vi "matched_filtering.vi"(8 "error in (no error)":errorcluster, 10 "input complex waveform":cluster{"t0":dbl, "dt":dbl, "Y":cdb[]}, 11 "Modulation Parameters In":T1={"RX Parameters"={"RX Oversample Factor"=4, "RX Sample Rate"=4000000.0, "Synchronization Options"={"Synchronization Method"=enum."Fixed Offset", "Symbol Timing Recovery Method "=enum."MT Allign To Ideal Symbols", "Fixed Offset"=0.0, "Frame Detection Method"=enum."", "Correct Frequency Offset"=FALSE}, "Channel Estimation/Equalization Parameters"={"Equalization Method"=enum."", "Channel Estimate Length"=0.0, "Equalizer Length"=0.0, "Equalizer Delay"=0.0}}, "TX/RX Shared Parameters"={"Modulation Type"=enum."OOK", "Packet Length"=128, "# of Iterations"=0.0, "Pulse Shaping Parameters"={"Pulse Shaping Filter"=enum."none", "Filter Length (symbols)"=32, "Filter Parameter"=0.8, "modulation type"=enum."FSK"}, "Header/Tail Control Information"={"Training Sequence Type"=enum."", "Zero Pad Length"=0.0}}}) -> (0 "error out":errorcluster, 2 "output complex waveform":cluster{"t0":dbl, "dt":dbl, "Y":cdb[]}, 3 "Modulation Parameters Out":T1={"RX Parameters"={"RX Oversample Factor"=4, "RX Sample Rate"=4000000.0, "Synchronization Options"={"Synchronization Method"=enum."Fixed Offset", "Symbol Timing Recovery Method "=enum."MT Allign To Ideal Symbols", "Fixed Offset"=0.0, "Frame Detection Method"=enum."", "Correct Frequency Offset"=FALSE}, "Channel Estimation/Equalization Parameters"={"Equalization Method"=enum."", "Channel Estimate Length"=0.0, "Equalizer Length"=0.0, "Equalizer Delay"=0.0}}, "TX/RX Shared Parameters"={"Modulation Type"=enum."OOK", "Packet Length"=128, "# of Iterations"=0.0, "Pulse Shaping Parameters"={"Pulse Shaping Filter"=enum."none", "Filter Length (symbols)"=32, "Filter Parameter"=0.8, "modulation type"=enum."FSK"}, "Header/Tail Control Information"={"Training Sequence Type"=enum."", "Zero Pad Length"=0.0}}})   [LabVIEW 2012]
uses:
  <vilib>/Analysis/2dsp.llb/1D Convolution (CDB).vi
  <vilib>/addons/Modulation/niDMT.lvlib
  <vilib>/Analysis/NI_AALPro.lvlib
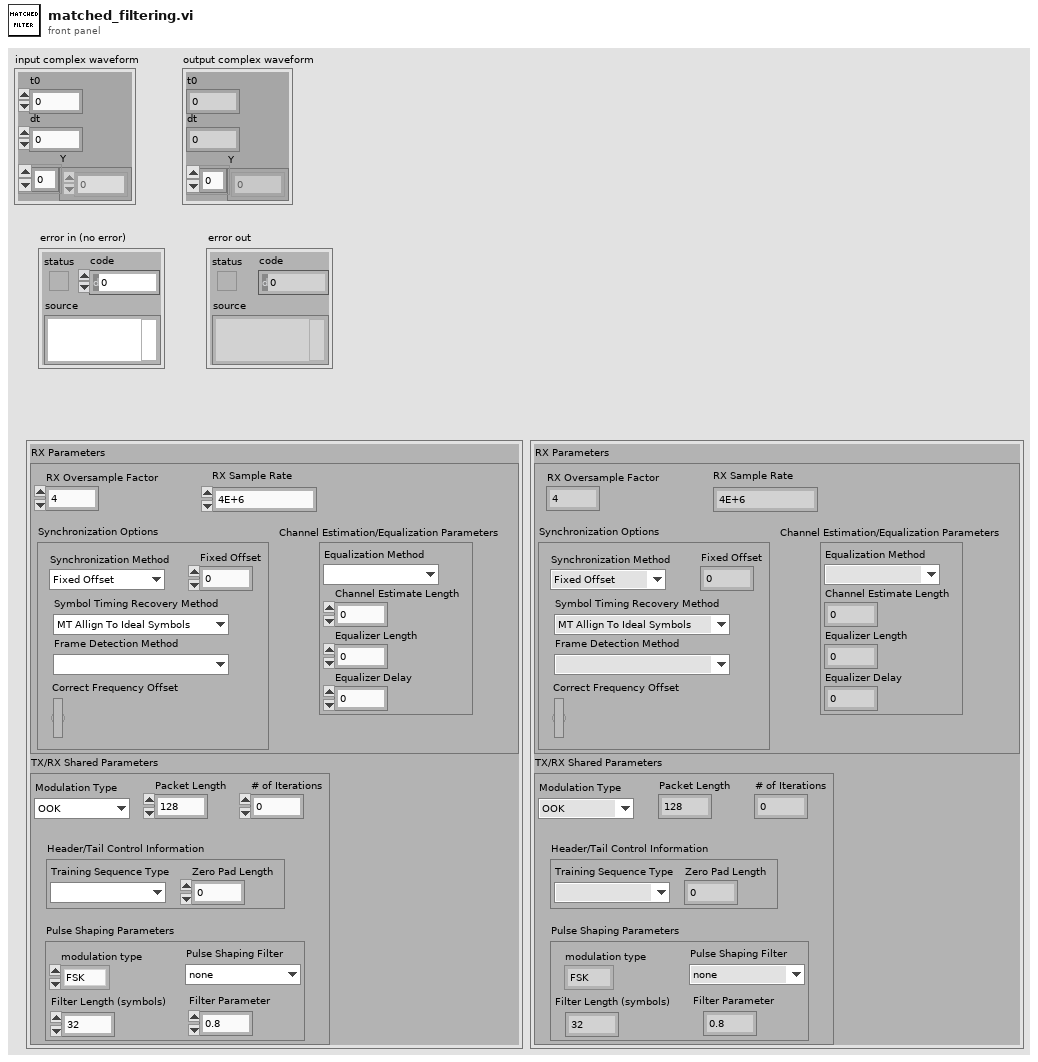
[diagram p1: front panel]
types:
  T1 = cluster{"RX Parameters":cluster{"RX Oversample Factor":i32, "RX Sample Rate":dbl, "Synchronization Options":cluster{"Synchronization Method":enum16{"Fixed Offset", "Timing Estimation", "Joint Timing and Channel Estimation"}, "Symbol Timing Recovery Method ":enum16{"MT Allign To Ideal Symbols", "Maximum Energy", "Early-Late Gate", "Gardner", "Fixed Offset"}, "Fixed Offset":dbl, "Frame Detection Method":enum16{""}, "Correct Frequency Offset":bool}, "Channel Estimation/Equalization Parameters":cluster{"Equalization Method":enum16{""}, "Channel Estimate Length":dbl, "Equalizer Length":dbl, "Equalizer Delay":dbl}}, "TX/RX Shared Parameters":cluster{"Modulation Type":enum16{"OOK", "FSK"}, "Packet Length":i32, "# of Iterations":dbl, "Pulse Shaping Parameters":cluster{"Pulse Shaping Filter":enum16{"none", "Raised Cosine", "Root Raised Cos", "Gaussian"}, "Filter Length (symbols)":i32, "Filter Parameter":dbl, "modulation type":enum16{"FSK", "PSK", "QAM", "MSK", "PAM", "ASK", "CPM"}}, "Header/Tail Control Information":cluster{"Training Sequence Type":enum16{""}, "Zero Pad Length":dbl}}}
  T2 = cluster{"Pulse Shaping Filter":enum16{"none", "Raised Cosine", "Root Raised Cos", "Gaussian"}, "Filter Length (symbols)":i32, "Filter Parameter":dbl, "modulation type":enum16{"FSK", "PSK", "QAM", "MSK", "PAM", "ASK", "CPM"}}
  T3 = enum16{"FSK", "PSK", "QAM", "MSK", "PAM", "ASK", "CPM"}
  T4 = enum16{"none", "Raised Cosine", "Root Raised Cos", "Gaussian"}
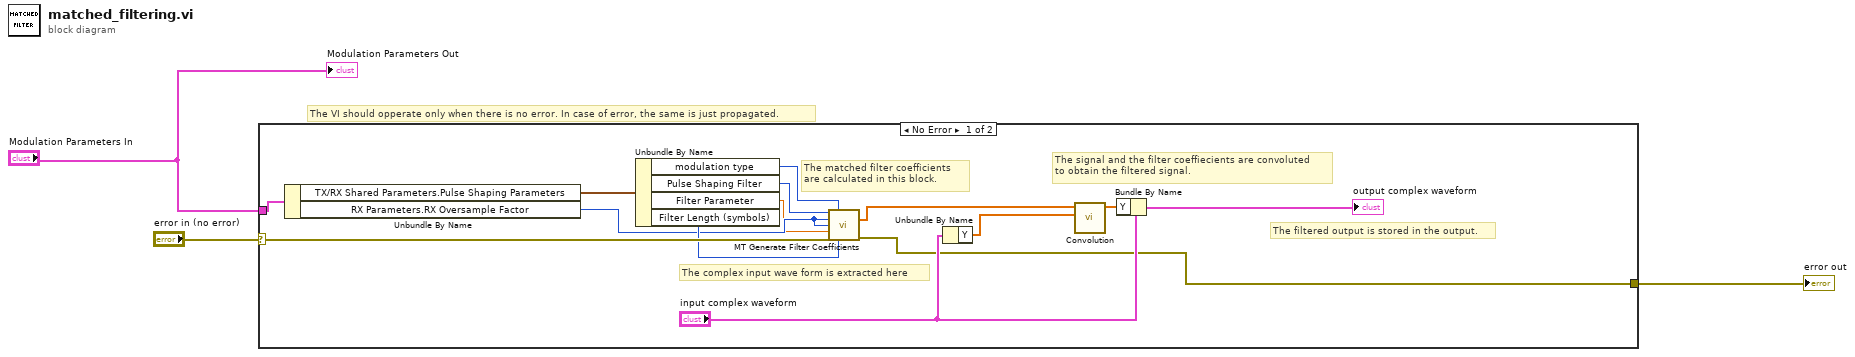
[diagram p0: block diagram]
diagram:
  # "The VI should opperate only when there is no error. In case of error, the same is just propagated."
  n1 = case shown="No Error" "error in (no error)" {
    selector: "error in (no error)" -> [w15 w18]
    tunnel: [w8 w18] -> w1
    tunnel: "Modulation Parameters In" -> [w17 _]
    frame No Error {
      # "The filtered output is stored in the output."
      # "The signal and the filter coeffiecients are convoluted\nto obtain the filtered signal."
      # "The complex input wave form is extracted here"
      # "The matched filter coefficients \nare calculated in this block."
      n2 = Unbundle By Name(w17) -> ("TX/RX Shared Parameters.Pulse Shaping Parameters"=w16:T2, "RX Parameters.RX Oversample Factor"=w7:i32)
      n3 = Unbundle By Name(w16) -> ("modulation type"=w5:T3, "Pulse Shaping Filter"=w4:T4, "Filter Parameter"=w6:dbl, "Filter Length (symbols)"=w14:i32)
      n4 = call <vilib>:"MT Generate Filter Coefficients.vi"("pulse shaping filter (none)"=w4, "modulation type"=w5, "pulse shaping samples per symbol (16)"=w7, "matched samples per symbol (16)"=w7, "filter parameter"=w6, "error in (no error)"=w15, "filter length (symbols)"=w14) -> ("matched filter coefficients"=w12:dbl[], "error out"=w8:errorcluster)  [unwired: 6 in, 1 out]
      n5 = Unbundle By Name("input complex waveform") -> ("Y"=w13:cdb[])
      n6 = call-poly <vilib>:"Convolution.vi"("Y"=w13, "X"=w12) -> ("X * Y"=w10:cdb[])  [unwired: 8 in, 1 out]
      n7 = Bundle By Name(cluster="input complex waveform", "Y"=w10) -> (→"output complex waveform":cluster{"t0":dbl, "dt":dbl, "Y":cdb[]})
    }
    frame Error {
    }
  }
  "error out" <- w1
  "Modulation Parameters Out" <- "Modulation Parameters In"
